vi "BRig_dataMTrig_warmup_OnOff.vi"() -> (2 "output_warmup_OnOff":i32)   [LabVIEW 2014]
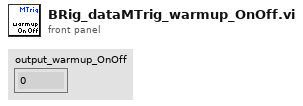
[diagram p1: front panel]
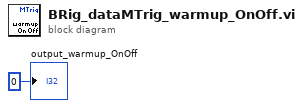
[diagram p0: block diagram]
diagram:
  "output_warmup_OnOff" <- 0 ("output_iBlock")
